vi "New Data Type Selector.vi"(4 "Size":T1, 6 "Position":T2, 8 "error in (no error)":errorcluster, 10 "Data Type Selector Return":refnum<user-event>, 11 "Data Type in":string) -> (0 "error out":errorcluster, 3 "Data Type Selector out":refnum<class "Data Type Selector.lvclass">)   [LabVIEW 2018, in "Data Type Selector.lvclass"]
uses:
  Data Type Selector.lvclass
  <vilib>/Utility/miscctls.llb/LVPointTypeDef.ctl
  <vilib>/Utility/miscctls.llb/LVBoundsTypeDef.ctl
  <vilib>/MGI/Panel Manager/Panel/Panel/Window/Dialog/Behavior.ctl
  <vilib>/MGI/Panel Manager/Panel/Window Position/Reference Position/Size/Absolute Size/Absolute Size.lvclass/Absolute Size.ctl
  <vilib>/MGI/Panel Manager/Panel/Window Position/Reference Position/Offset/Absolute Offset/Absolute Offset.lvclass/Absolute Offset.ctl
  Data Type Selector.lvclass/Data Type Selector.ctl
  <vilib>/MGI/Panel Manager/Panel/Window Position/Reference Position/Size/Absolute Size/Absolute Size.vi
  <vilib>/MGI/Panel Manager/Panel/Window Position/Reference Position/Offset/Absolute Offset/Absolute Offset.vi
  <vilib>/MGI/Panel Manager/Panel/Window Position/Reference Position/Size/Absolute Size/Absolute Size.lvclass
  C:/Program Files (x86)/National Instruments/LabVIEW 2018/vi.lib/MGI/Panel Manager/Panel/Window Position/Reference Position/Size/Size.lvclass
  <vilib>/MGI/Panel Manager/Panel/Window Position/Reference Position/Offset/Absolute Offset/Absolute Offset.lvclass
  C:/Program Files (x86)/National Instruments/LabVIEW 2018/vi.lib/MGI/Panel Manager/Panel/Window Position/Reference Position/Offset/Offset.lvclass
  <vilib>/MGI/Panel Manager/Panel/Window Position/Reference Position/Ref Display/Ref Display.lvclass
  C:/Program Files (x86)/National Instruments/LabVIEW 2018/vi.lib/MGI/Panel Manager/Panel/Window Position/Window Position.lvclass
  <vilib>/MGI/Panel Manager/Panel/Panel/Window/Dialog/Dialog.lvclass
  C:/Program Files (x86)/National Instruments/LabVIEW 2018/vi.lib/MGI/Panel Manager/Panel/Panel/Panel.lvclass
  <vilib>/MGI/Panel Manager/Panel/Window Position/Reference Position/Ref Display/Ref Display.vi
  <vilib>/MGI/Panel Manager/Panel/Panel/Window/Dialog/Dialog.vi
  <vilib>/MGI/Panel Manager/Panel/Panel.lvlib
  C:/Program Files (x86)/National Instruments/LabVIEW 2018/vi.lib/MGI/Panel Manager/Panel/Window Position/Reference Position/Reference Position.lvclass
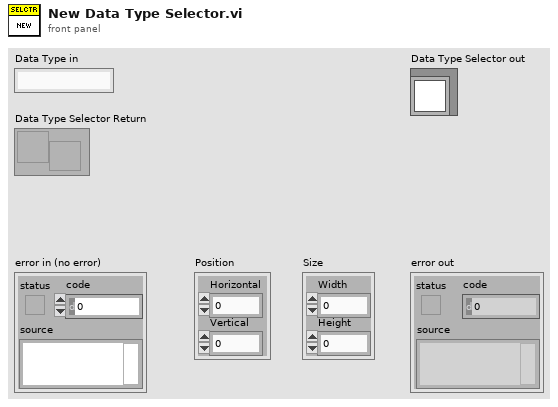
[diagram p1: front panel]
types:
  T1 = typedef "LVBoundsTypeDef.ctl" = cluster{"Width":u32, "Height":u32}
  T2 = typedef "LVPointTypeDef.ctl" = cluster{"Horizontal":i16, "Vertical":i16}
  T3 = typedef "Panel.lvlib/Dialog.lvclass/Behavior.ctl" = enum32{"Floating", "Floating/Auto-Hide", "Modal"}
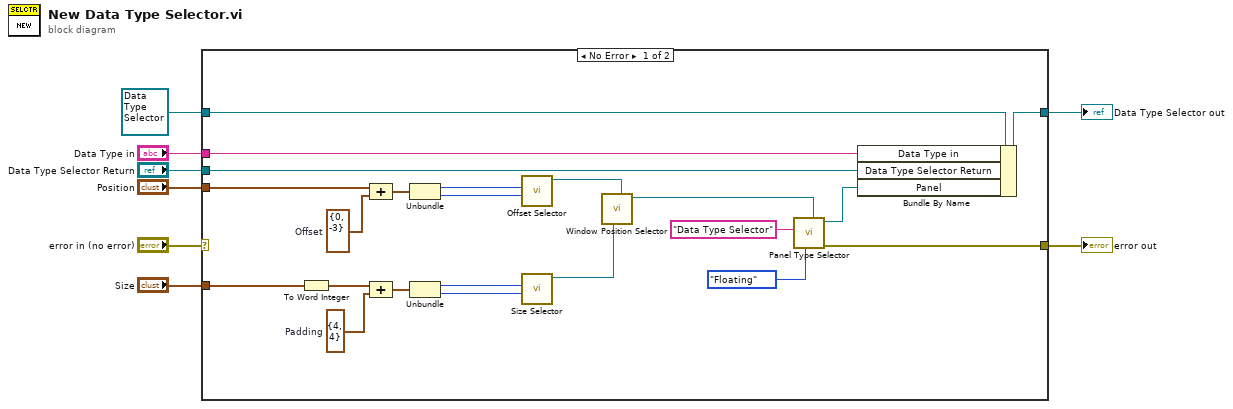
[diagram p0: block diagram]
diagram:
  n1 = case shown="No Error" "error in (no error)" {
    selector: "error in (no error)" -> [_ w32]
    tunnel: [w29 w32] -> w7
    tunnel: [w24 w31] -> w5
    tunnel: refnum<class "Data Type Selector.lvclass"> refnum ("Data Type Selector in") -> [w25 w31]
    tunnel: "Data Type in" -> [w28 _]
    tunnel: "Data Type Selector Return" -> [w27 _]
    tunnel: "Position" -> [w12 _]
    tunnel: "Size" -> [w21 _]
    frame No Error {
      w10 = cluster{"Width":i16, "Height":i16} {"Width"=0, "Height"=-3}  # Offset
      w16 = cluster{"Width":i16, "Height":i16} {"Width"=4, "Height"=4}  # Padding
      n2 = To Word Integer(number=w21) -> (16bit integer=w18:cluster{"Width":i16, "Height":i16})
      n3 = Compound Arithmetic op=ADD(w12, w10) -> (w11:T2)
      n4 = Compound Arithmetic op=ADD(w18, w16) -> (w17:cluster{"Width":i16, "Height":i16})
      n5 = Unbundle(w11) -> ("Horizontal"=w14:i16, "Vertical"=w13:i16)
      n6 = Unbundle(w17) -> ("Width"=w20:i16, "Height"=w19:i16)
      n7 = call-poly <vilib>:"Offset Selector.vi"("Vertical"=w13, "Horizontal"=w14) -> ("Absolute Offset Out"=w22:refnum<class "Absolute Offset.lvclass">)  [unwired: 8 in, 1 out]
      n8 = call-poly <vilib>:"Size Selector.vi"("Height"=w19, "Width"=w20) -> ("Absolute Size out"=w23:refnum<class "Absolute Size.lvclass">)  [unwired: 8 in, 1 out]
      n9 = call-poly <vilib>:"Window Position Selector.vi"("Offset"=w22, "Size"=w23) -> ("Ref Display out"=w15:refnum<class "Ref Display.lvclass">)  [unwired: 8 in, 1 out]
      n10 = call-poly <vilib>:"Panel Type Selector.vi"("Window Position (Center in Top Level)"=w15, "Behavior (Modal)"=Behavior."Floating", "Default Title"="Data Type Selector") -> ("Error Out"=w29:errorcluster, "Dialog out"=w26:refnum<class "Dialog.lvclass">)  [unwired: 7 in]
      n11 = Bundle By Name(cluster=w25, "Data Type in"=w28, "Data Type Selector Return"=w27, "Panel"=w26) -> (w24:refnum<class "Data Type Selector.lvclass">)
    }
    frame Error {
    }
  }
  "error out" <- w7
  "Data Type Selector out" <- w5
